vi "Camera_AcquireMultipleImages.vi"(3 "error in":errorcluster, 4 "Number of Images":i32=5) -> (0 "error out":errorcluster, 1 "Images Out":T1[](array[typedef]))   [LabVIEW 2009, in "Camera.lvlib"]
uses:
  Camera.lvlib
  <vilib>/vision/Image Controls.llb/IMAQ Image.ctl
panel:
  out "Image Out":T1(plugin-control)
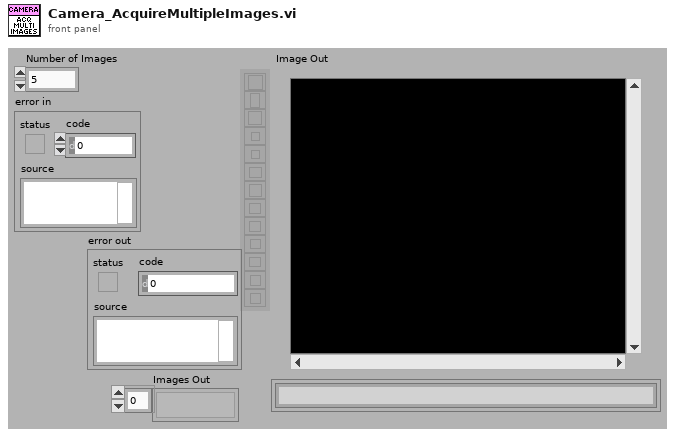
[diagram p1: front panel]
types:
  T1 = typedef "IMAQ Image.ctl" = refnum<image>
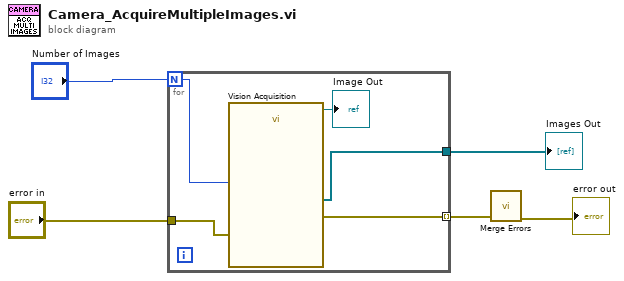
[diagram p0: block diagram]
diagram:
  n1 = for {
    N: "Number of Images" -> [w9]
    tunnel: "error in" -> [w8]
    tunnel: [w7] -> w3 mode=indexing
    tunnel: [w6] -> w1
    n2 = call "Vision Acquisition"("Number of Images"=w9, "error in"=w8) -> ("Image Out"=→"Image Out":T1, "All Images Out"=w6:refnum<image>[], "error out"=w7:errorcluster)  [unwired: 23 in]
  }
  "Images Out" <- w1
  n3 = call <vilib>:"Merge Errors.vi"("error array in"=w3) -> ("error out"=→"error out":errorcluster)  [unwired: 6 in]
